vi "Splash Screen User Event LV2.vi"(6 "Command":T2=enum."Generate", 8 "error in (no error)":errorcluster, 11 "Splash Screen":T1) -> (0 "error out":errorcluster, 3 "Splash Screen Event":refnum<user-event>)   [LabVIEW 2014, in "SLL Splash Screen.lvlib"]
uses:
  SLL Splash Screen.lvlib
  _Typedefs/User Event LV2 Command.ctl
  _Typedefs/Splash Screen Data.ctl
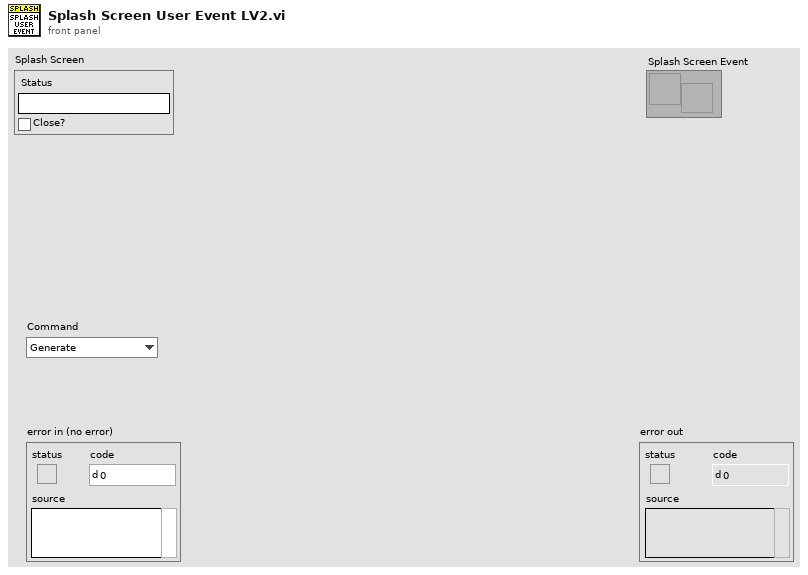
[diagram p1: front panel]
types:
  T1 = typedef "SLL Splash Screen.lvlib/Splash Screen Data.ctl" = cluster{"Status":string, "Close?":bool}
  T2 = typedef "SLL Splash Screen.lvlib/User Event LV2 Command.ctl" = enum16{"Create", "Generate", "Delete"}
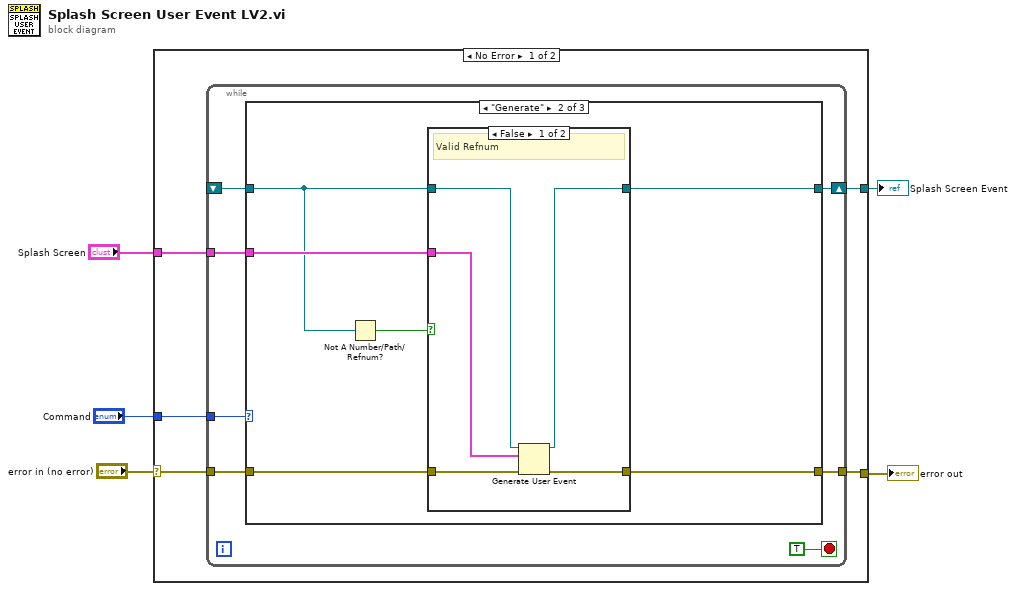
[diagram p0: block diagram]
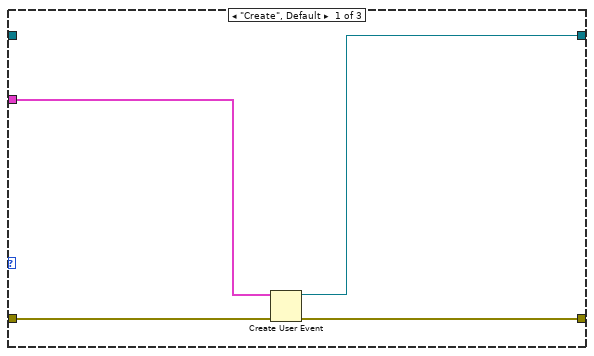
[diagram p2: hidden frame]
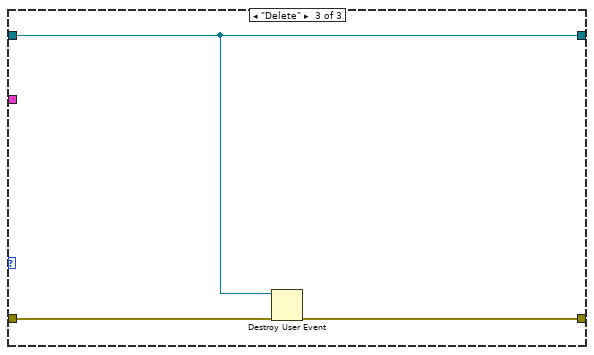
[diagram p4: hidden frame]
diagram:
  n1 = case shown="No Error" "error in (no error)" {
    selector: "error in (no error)" -> [w8 w38]
    tunnel: [w7 w38] -> w4
    tunnel: "Command" -> [w10 _]
    tunnel: "Splash Screen" -> [w9 _]
    tunnel: [w6 _] -> w1
    frame No Error {
      n2 = while {
        tunnel: w10 -> [w16]
        tunnel: w9 -> [w15]
        tunnel: w8 -> [w14]
        tunnel: [w13] -> w7
        shift-right: [w12] -> w6
        shift-left: _ -> [w11]
        stop <- TRUE stop-if-true
        n3 = case shown="\"Generate\"" w16 {
          tunnel: w15 -> [w19 w24 _]
          tunnel: w14 -> [w21 w27 w37]
          tunnel: [w20 w26 w36] -> w13
          tunnel: [w18 w25 w35] -> w12
          tunnel: w11 -> [_ w23 w35]
          frame "Create", Default {
            n4 = Create User Event(user event datatype=w19, error in=w21) -> (user event=w18:refnum<user-event>, error out=w20:errorcluster)
          }
          frame "Generate" {
            n5 = Not A Number/Path/Refnum?(number/path/refnum=w23) -> (NaN/Path/Refnum?=w22:bool)
            n6 = case shown="False" w22 {
              tunnel: w27 -> [w32 w33]
              tunnel: [w31 w33] -> w26
              tunnel: [w30 w34] -> w25
              tunnel: w24 -> [w29 _]
              tunnel: w23 -> [w28 w34]
              frame False {
                # "Valid Refnum"
                n7 = Generate User Event(user event=w28, event data cluster=w29, error in=w32) -> (user event out=w30:refnum<user-event>, error out=w31:errorcluster)  [unwired: 1 in]
              }
              frame True {
                # "Invalid Refnum"
              }
            }
          }
          frame "Delete" {
            n8 = Destroy User Event(user event=w35, error in=w37) -> (error out=w36:errorcluster)
          }
        }
      }
    }
    frame Error {
    }
  }
  "error out" <- w4
  "Splash Screen Event" <- w1
